vi "20211015_HW01.vi"() -> ()   [LabVIEW 2019]
panel:
  in  "Next Line":bool
  out "Output String":string
  in  "Input String":string="《倚天屠龍記》為香港作家金庸所著武俠小說「射鵰三部曲」之一。男主角為張無忌，女主角則為趙敏，為其三部曲之最後一部。"
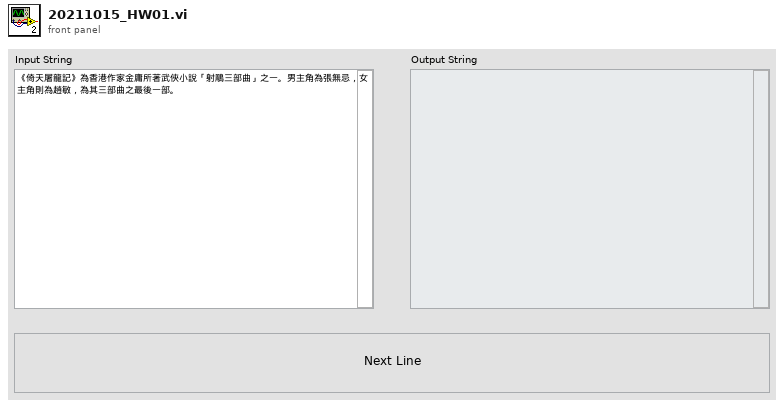
[diagram p1: front panel]
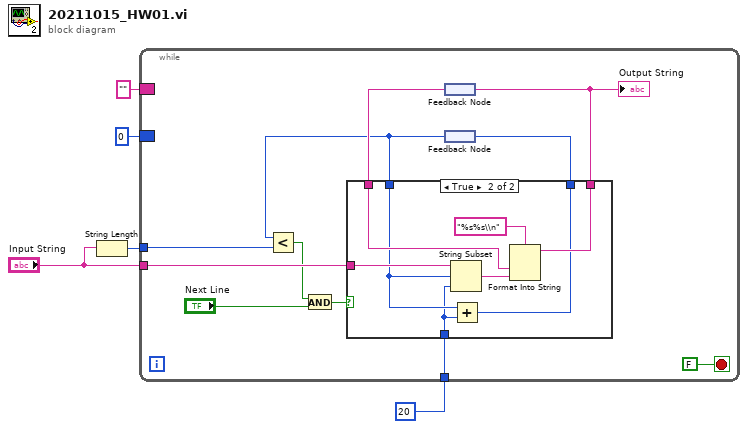
[diagram p0: block diagram]
diagram:
  n1 = String Length(string="Input String") -> (length=w1:i32)
  n2 = while {
    tunnel: "Input String" -> [w16]
    border: "" -> [_]
    border: 0 ("offset (0)") -> [_]
    tunnel: 20 ("length (rest)") -> [w11]
    tunnel: w1 -> [w9]
    stop <- FALSE stop-if-true
    n3 = feedback #1() -> (w14:string)
    n4 = feedback #2() -> (w10:i32)
    n5 = Less?(x=w10, y=w9) -> (x < y?=w7:bool)
    n6 = And(x=w7, y="Next Line") -> (x .and. y?=w6:bool)
    n7 = case shown="True" w6 {
      tunnel: w16 -> [_ w26]
      tunnel: w10 -> [w18 w21]
      tunnel: [w18 w19] -> w15
      tunnel: [w17 w24] -> w13
      tunnel: w14 -> [w17 w22]
      tunnel: w11 -> [_ w20]
      frame False {
      }
      frame True {
        n8 = String Subset(string=w26, offset (0)=w21, length (rest)=w20) -> (substring=w23:string)
        n9 = Add(x=w21, y=w20) -> (x+y=w19:i32)
        n10 = Format Into String(format string="%s%s\\n", w22, w23) -> (resulting string=w24:string)  [unwired: 2 in, 1 out]
      }
    }
    "Output String" <- w13
    n11 = feedback-in #1(w13) -> ()
    n12 = feedback-in #2(w15) -> ()
  }
